vi "BRig_RT__Case_Exp__State_initTrial2__v17.vi"(0 "input_dataCurrent":u16[](array[numeric]), 1 "input_dataTrial":u16[][](array[numeric]), 3 "input_dataExp":u16[](array[numeric]), 6 "input_dataBlock":u16[][](array[numeric]), 8 "input_dataLC":u16[](array[numeric])) -> (7 "output_L_Wrong_Laser_l2":bool, 9 "output_L_Wrong_Event_l2":bool, 10 "output_L_Power_l1":dbl, 11 "output_L_Reward_Laser_l2":bool, 12 "output_L_Power_l2":dbl, 13 "output_L_Reward_Event_l2":bool, 14 "output_dataCurrent":u16[](array[numeric]), 15 "output_dataTrial":u16[][](array[numeric]), 16 "output_L_Reward_Event_l1":bool, 17 "output_L_Reward_Laser_l1":bool, 18 "output_L_Wrong_Event_l1":bool, 19 "output_L_Wrong_Laser_l1":bool)   [LabVIEW 2014]
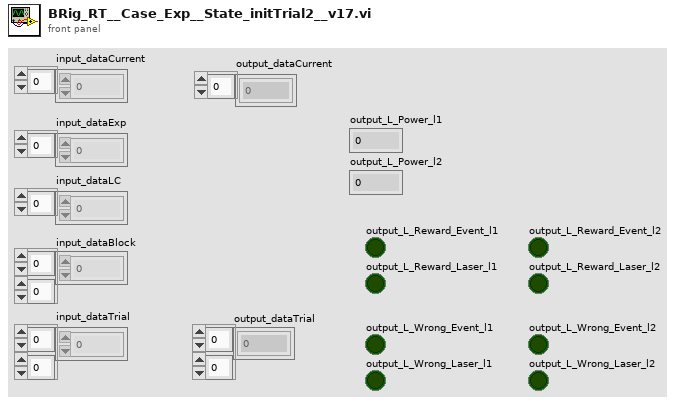
[diagram p1: front panel]
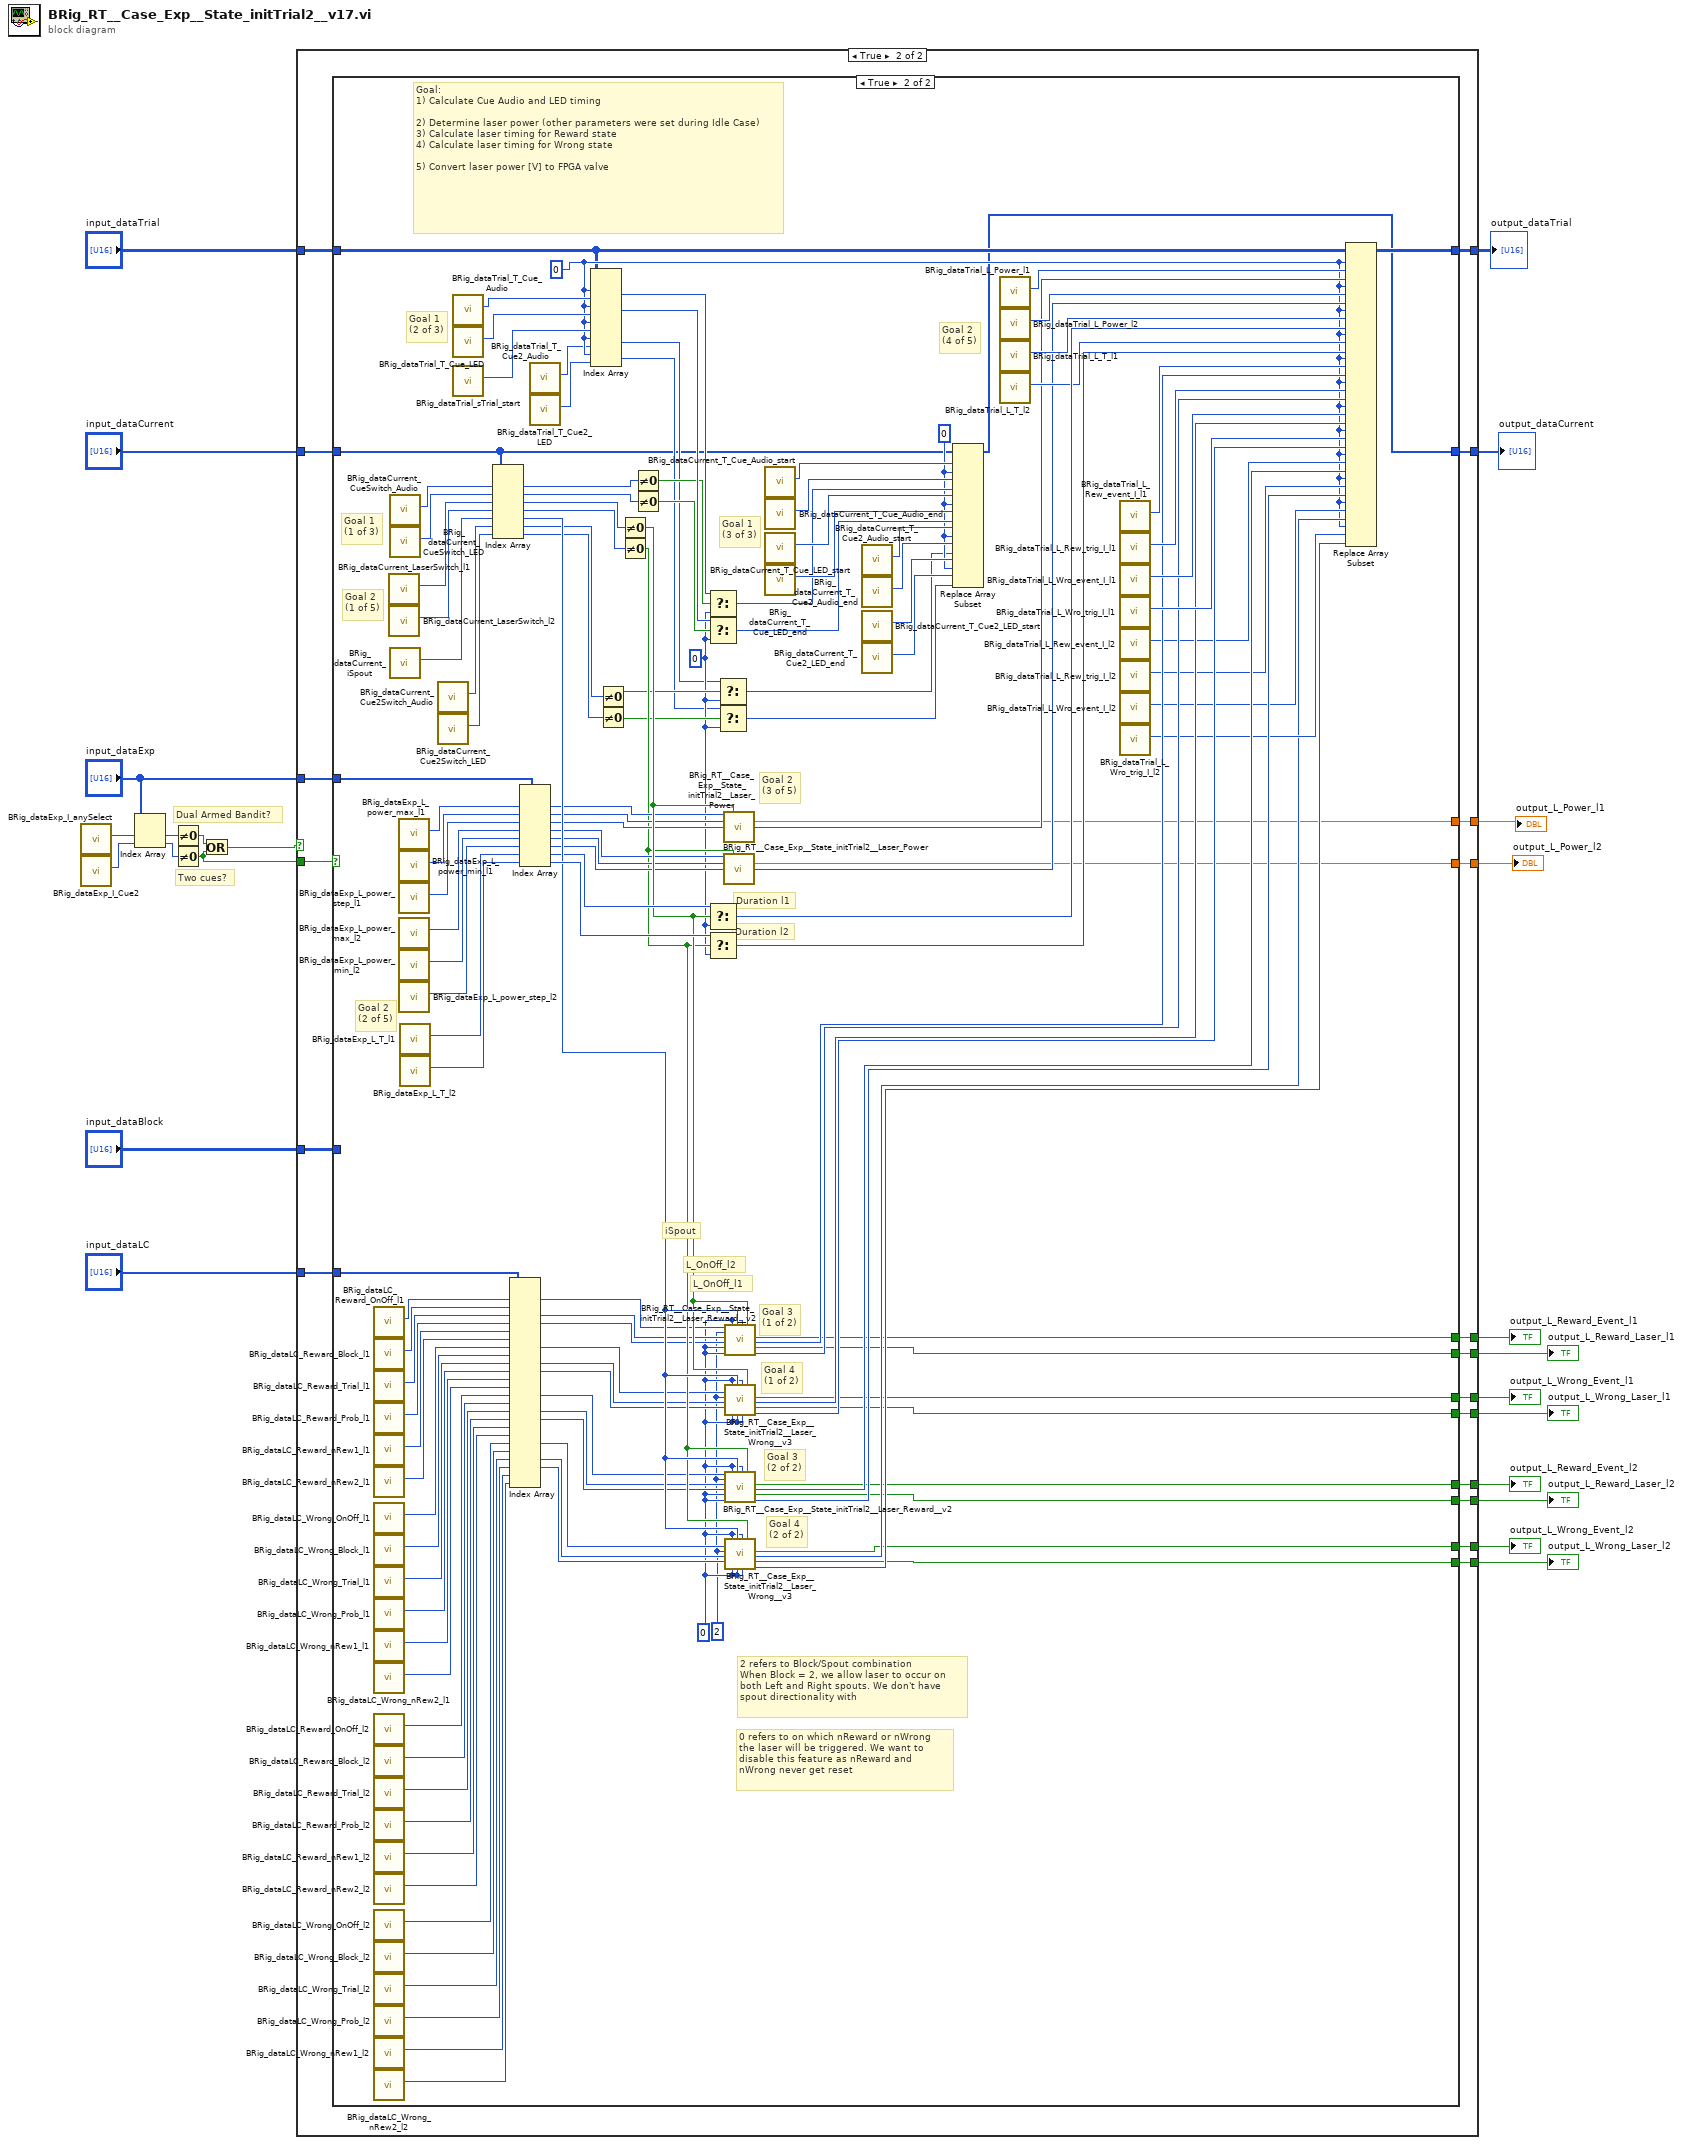
[diagram p0: block diagram]
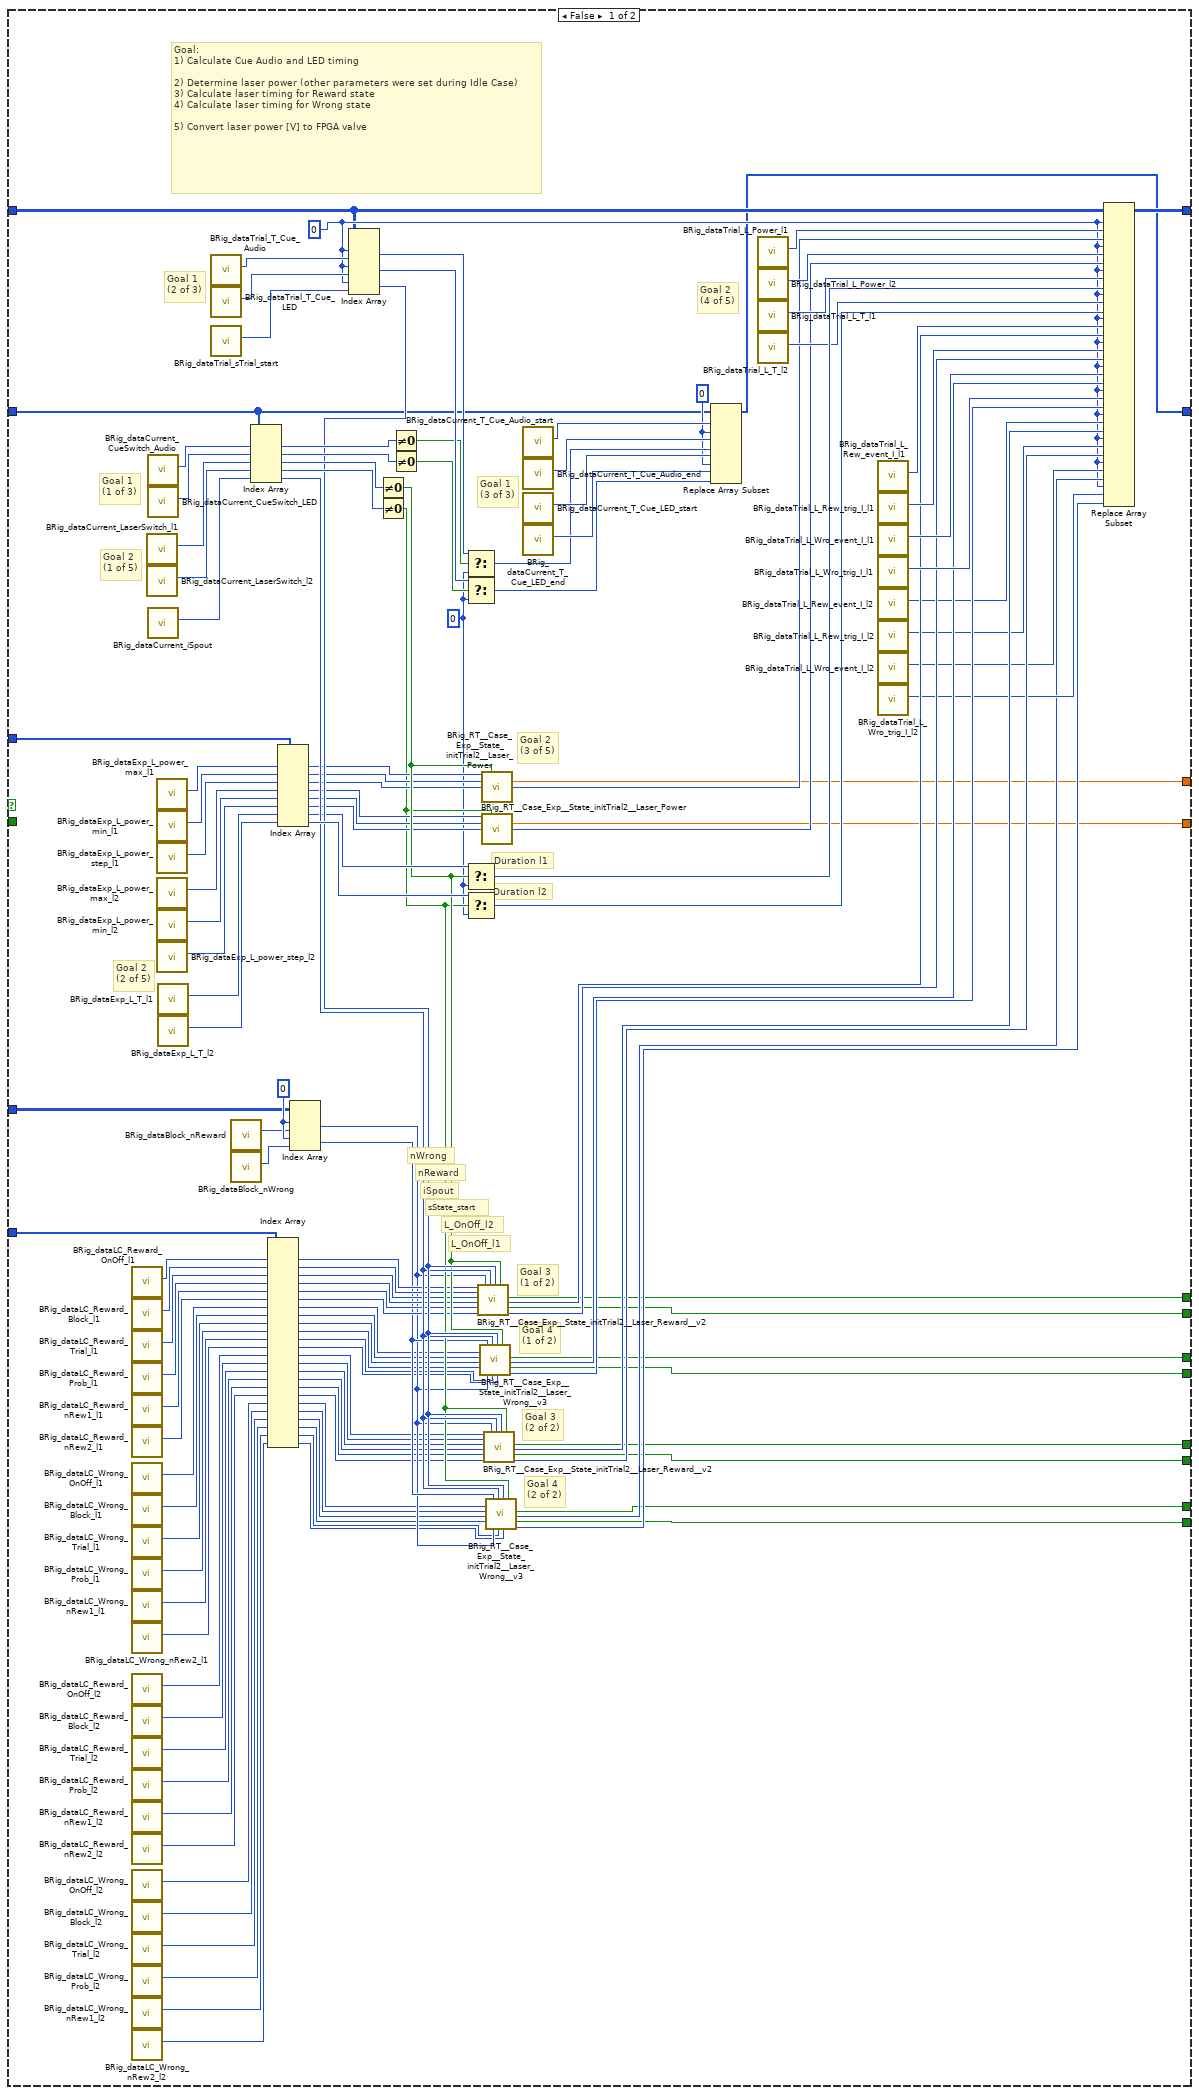
[diagram p2: hidden frame]
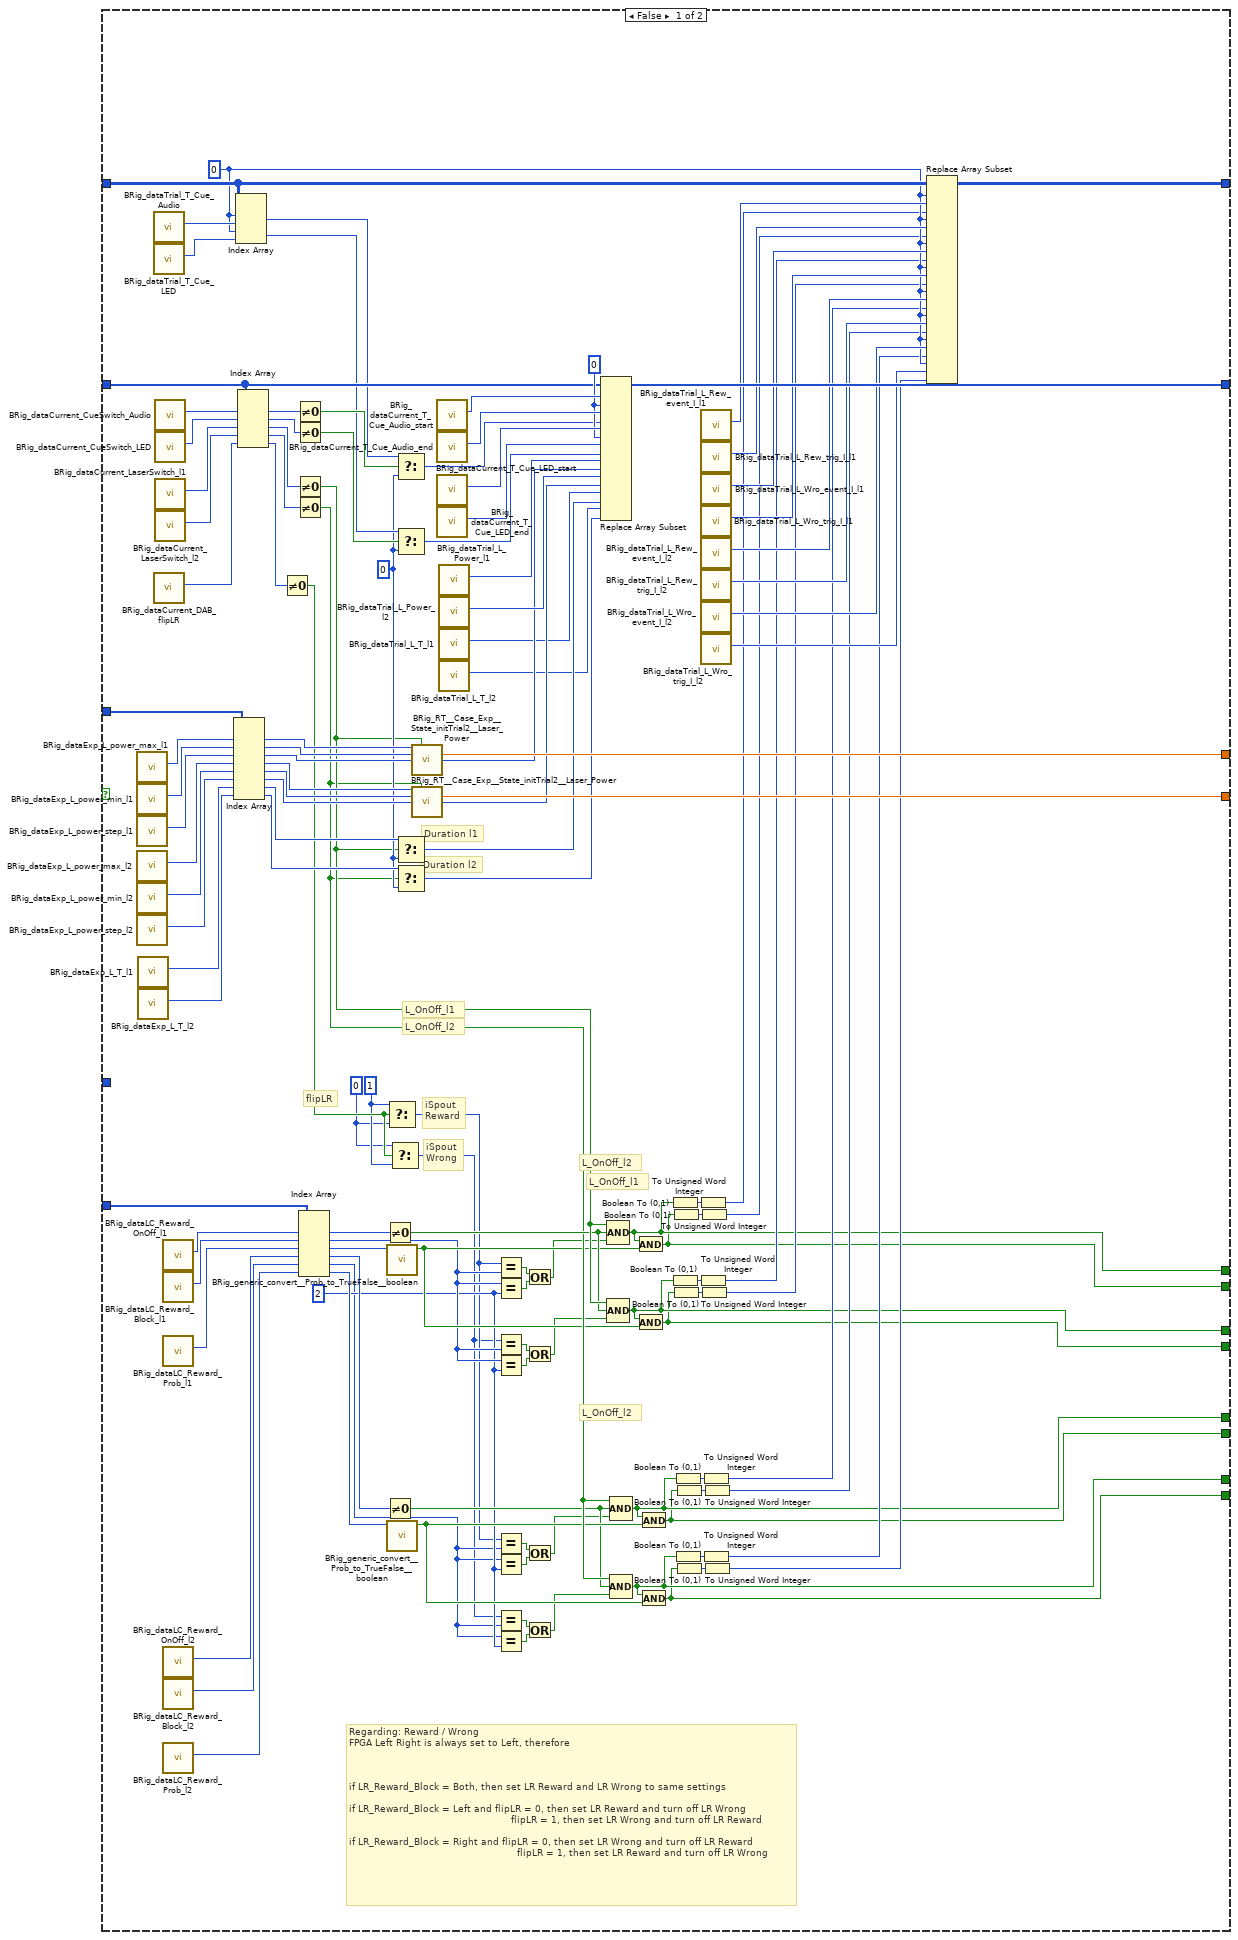
[diagram p3: hidden frame]
diagram:
  # "Two cues?"
  # "Dual Armed Bandit?"
  n1 = call "BRig_dataExp_I_anySelect.vi"() -> ("output_I_anySelect"=w9:i32)  [unwired: 11 in]
  n2 = call "BRig_dataExp_I_Cue2.vi"() -> ("output_I_Cue2"=w7:i32)  [unwired: 11 in]
  n3 = Index Array(array="input_dataExp", index #1=w9, index #2=w7) -> (element #1=w8:u16, element #2=w6:u16)
  n4 = Not Equal To 0?(x=w8) -> (x != 0?=w5:bool)
  n5 = Not Equal To 0?(x=w6) -> (x != 0?=w3:bool)
  n6 = Or(x=w5, y=w3) -> (x .or. y?=w4:bool)
  n7 = case shown="True" w4 {
    tunnel: [w41 w174] -> w24
    tunnel: "input_dataTrial" -> [w40 w175]
    tunnel: "input_dataCurrent" -> [w39 w181]
    tunnel: "input_dataExp" -> [w38 w179]
    tunnel: "input_dataBlock" -> [w37 w164]
    tunnel: "input_dataLC" -> [w36 w176]
    tunnel: [w35 w173] -> w19
    tunnel: [w34 w172] -> w18
    tunnel: [w33 w171] -> w17
    tunnel: [w32 w170] -> w16
    tunnel: [w31 w169] -> w15
    tunnel: [w30 w168] -> w14
    tunnel: [w29 w167] -> w13
    tunnel: [w28 w166] -> w12
    tunnel: [w27 w177] -> w11
    tunnel: [w26 w178] -> w10
    tunnel: [w25 w180] -> w1
    tunnel: w3 -> [_ w165]
    frame False {
      w89 = 0 ("disabled index (row)")
      w93 = 0
      w92 = u16 0 ("f")
      w91 = u16 0 ("new element/subarray")
      # "nWrong"
      # "nReward"
      # "L_OnOff_l2"
      # "Goal 2\n(3 of 5)"
      # "Goal 4\n(2 of 2)"
      # "Goal 4\n(1 of 2)"
      # "Goal 3\n(2 of 2)"
      # "Goal 3\n(1 of 2)"
      # "L_OnOff_l1"
      # "sState_start"
      # "iSpout"
      # "Goal 2\n(4 of 5)"
      # "Goal 2\n(2 of 5)"
      # "Duration l2"
      # "Duration l1"
      # "Goal 2\n(1 of 5)"
      # "Goal 1\n(3 of 3)"
      # "Goal 1\n(2 of 3)"
      # "Goal 1\n(1 of 3)"
      # "Goal:\n1) Calculate Cue Audio and LED timing\n\n2) Determine laser power (other parameters were set during Idle Case)\n3) Calculate laser timing for Reward state\n4) Calculate laser timing for Wrong state\n\n5) Convert laser power [V] to FPGA valve"
      n8 = call "BRig_dataLC_Reward_OnOff_l1.vi"() -> ("output_Reward_OnOff"=w130:i32)  [unwired: 11 in]
      n9 = call "BRig_dataLC_Reward_Block_l1.vi"() -> ("output_Reward_Block"=w129:i32)  [unwired: 11 in]
      n10 = call "BRig_dataLC_Reward_Trial_l1.vi"() -> ("output_Reward_Trial"=w128:i32)  [unwired: 11 in]
      n11 = call "BRig_dataLC_Reward_Prob_l1.vi"() -> ("output_Reward_Prob"=w127:i32)  [unwired: 11 in]
      n12 = call "BRig_dataLC_Reward_nRew1_l1.vi"() -> ("output_Reward_nRew1_l1"=w83:i32)  [unwired: 11 in]
      n13 = call "BRig_dataLC_Reward_nRew2_l1.vi"() -> ("output_Reward_nRew2_l1"=w82:i32)  [unwired: 11 in]
      n14 = call "BRig_dataLC_Wrong_OnOff_l1.vi"() -> ("output_Wrong_OnOff"=w79:i32)  [unwired: 11 in]
      n15 = call "BRig_dataLC_Wrong_Block_l1.vi"() -> ("output_Wrong_Block"=w78:i32)  [unwired: 11 in]
      n16 = call "BRig_dataLC_Wrong_Trial_l1.vi"() -> ("output_Wrong_Trial"=w77:i32)  [unwired: 11 in]
      n17 = call "BRig_dataLC_Wrong_Prob_l1.vi"() -> ("output_Wrong_Prob"=w76:i32)  [unwired: 11 in]
      n18 = call "BRig_dataLC_Wrong_nRew1_l1.vi"() -> ("output_Wrong_nRew1_l1"=w57:i32)  [unwired: 11 in]
      n19 = call "BRig_dataLC_Wrong_nRew2_l1.vi"() -> ("output_Wrong_nRew2_l1"=w56:i32)  [unwired: 11 in]
      n20 = call "BRig_dataLC_Reward_OnOff_l2.vi"() -> ("output_Reward_OnOff_l2"=w64:i32)  [unwired: 11 in]
      n21 = call "BRig_dataLC_Reward_Block_l2.vi"() -> ("output_Reward_Block_l2"=w65:i32)  [unwired: 11 in]
      n22 = call "BRig_dataLC_Reward_Trial_l2.vi"() -> ("output_Reward_Trial_l2"=w66:i32)  [unwired: 11 in]
      n23 = call "BRig_dataLC_Reward_Prob_l2.vi"() -> ("output_Reward_Prob_l2"=w67:i32)  [unwired: 11 in]
      n24 = call "BRig_dataLC_Reward_nRew1_l2.vi"() -> ("output_Reward_nRew1_l2"=w68:i32)  [unwired: 11 in]
      n25 = call "BRig_dataLC_Reward_nRew2_l2.vi"() -> ("output_Reward_nRew2_l2"=w69:i32)  [unwired: 11 in]
      n26 = call "BRig_dataLC_Wrong_OnOff_l2.vi"() -> ("output_Wrong_OnOff_l2"=w70:i32)  [unwired: 11 in]
      n27 = call "BRig_dataLC_Wrong_Block_l2.vi"() -> ("output_Wrong_Block_l2"=w71:i32)  [unwired: 11 in]
      n28 = call "BRig_dataLC_Wrong_Trial_l2.vi"() -> ("output_Wrong_Trial_l2"=w72:i32)  [unwired: 11 in]
      n29 = call "BRig_dataLC_Wrong_Prob_l2.vi"() -> ("output_Wrong_Prob_l2"=w73:i32)  [unwired: 11 in]
      n30 = call "BRig_dataLC_Wrong_nRew1_l2.vi"() -> ("output_Wrong_nRew1_l2"=w49:i32)  [unwired: 11 in]
      n31 = call "BRig_dataLC_Wrong_nRew2_l2.vi"() -> ("output_Wrong_nRew2_l2"=w48:i32)  [unwired: 11 in]
      n32 = call "BRig_dataCurrent_LaserSwitch_l1.vi"() -> ("output_LaserSwitch_l1"=w149:i32)  [unwired: 11 in]
      n33 = call "BRig_dataCurrent_LaserSwitch_l2.vi"() -> ("output_LaserSwitch_l2"=w148:i32)  [unwired: 11 in]
      n34 = call "BRig_dataCurrent_CueSwitch_Audio.vi"() -> ("output_CueSwitch_Audio"=w163:i32)  [unwired: 11 in]
      n35 = call "BRig_dataCurrent_CueSwitch_LED.vi"() -> ("output_CueSwitch_LED"=w162:i32)  [unwired: 11 in]
      n36 = call "BRig_dataCurrent_iSpout.vi"() -> ("output_iSpout"=w124:i32)  [unwired: 11 in]
      n37 = call "BRig_dataExp_L_power_max_l1.vi"() -> ("output_L_power_max_l1"=w147:i32)  [unwired: 11 in]
      n38 = call "BRig_dataExp_L_power_min_l1.vi"() -> ("output_L_power_min_l1"=w146:i32)  [unwired: 11 in]
      n39 = call "BRig_dataExp_L_power_step_l1.vi"() -> ("output_L_power_step_l1"=w145:i32)  [unwired: 11 in]
      n40 = call "BRig_dataExp_L_power_max_l2.vi"() -> ("output_L_power_max_l2"=w144:i32)  [unwired: 11 in]
      n41 = call "BRig_dataExp_L_power_min_l2.vi"() -> ("output_L_power_min_l2"=w143:i32)  [unwired: 11 in]
      n42 = call "BRig_dataExp_L_power_step_l2.vi"() -> ("output_L_power_step_l2"=w142:i32)  [unwired: 11 in]
      n43 = call "BRig_dataExp_L_T_l1.vi"() -> ("output_L_T_l1"=w141:i32)  [unwired: 11 in]
      n44 = call "BRig_dataExp_L_T_l2.vi"() -> ("output_L_T_l2"=w140:i32)  [unwired: 11 in]
      n45 = call "BRig_dataTrial_T_Cue_Audio.vi"() -> ("output_T_Cue_Audio"=w154:i32)  [unwired: 11 in]
      n46 = call "BRig_dataTrial_T_Cue_LED.vi"() -> ("output_T_Cue_LED"=w153:i32)  [unwired: 11 in]
      n47 = call "BRig_dataTrial_sTrial_start.vi"() -> ("output_sTrial_start"=w123:i32)  [unwired: 11 in]
      n48 = call "BRig_dataBlock_nReward.vi"() -> ("output_nReward"=w88:i32)  [unwired: 11 in]
      n49 = call "BRig_dataBlock_nWrong.vi"() -> ("output_nWrong"=w90:i32)  [unwired: 11 in]
      n50 = Index Array(array=w39, index #1=w163, index #2=w162, index #3=w149, index #4=w148, index #5=w124) -> (element #1=w157:u16, element #2=w156:u16, element #3=w126:u16, element #4=w125:u16, element #5=w121:u16)
      n51 = Index Array(array=w36, index #1=w130, index #2=w129, index #3=w128, index #4=w127, index #5=w83, index #6=w82, index #7=w79, index #8=w78, index #9=w77, index #10=w76, index #11=w57, index #12=w56, index #13=w64, index #14=w65, index #15=w66, index #16=w67, index #17=w68, index #18=w69, index #19=w70, index #20=w71, index #21=w72, index #22=w73, index #23=w49, index #24=w48) -> (element #1=w87:u16, element #2=w86:u16, element #3=w85:u16, element #4=w84:u16, element #5=w81:u16, element #6=w80:u16, element #7=w55:u16, element #8=w54:u16, element #9=w53:u16, element #10=w52:u16, element #11=w51:u16, element #12=w50:u16, element #13=w58:u16, element #14=w59:u16, element #15=w60:u16, element #16=w61:u16, element #17=w62:u16, element #18=w63:u16, element #19=w47:u16, element #20=w46:u16, element #21=w45:u16, element #22=w44:u16, element #23=w43:u16, element #24=w42:u16)
      n52 = Index Array(array=w38, index #1=w147, index #2=w146, index #3=w145, index #4=w144, index #5=w143, index #6=w142, index #7=w141, index #8=w140) -> (element #1=w102:u16, element #2=w101:u16, element #3=w100:u16, element #4=w98:u16, element #5=w97:u16, element #6=w96:u16, element #7=w104:u16, element #8=w137:u16)
      n53 = Index Array(array=w37, index (row) #1=w89, index (col) #1=w88, index (row) #2=w89, index (col) #2=w90) -> (element #1=w74:u16, element #2=w75:u16)
      n54 = Index Array(array=w40, index (row) #1=w93, index (col) #1=w154, index (row) #2=w93, index (col) #2=w153, index (row) #3=w93, index (col) #3=w123) -> (element #1=w152:u16, element #2=w151:u16, element #3=w122:u16)
      n55 = Not Equal To 0?(x=w126) -> (x != 0?=w103:bool)
      n56 = Not Equal To 0?(x=w125) -> (x != 0?=w95:bool)
      n57 = Not Equal To 0?(x=w157) -> (x != 0?=w139:bool)
      n58 = Not Equal To 0?(x=w156) -> (x != 0?=w138:bool)
      n59 = Select(t=w152, s=w139, f=w92) -> (s? t:f=w155:u16)
      n60 = Select(t=w151, s=w138, f=w92) -> (s? t:f=w150:u16)
      n61 = Select(t=w104, s=w103, f=w92) -> (s? t:f=w133:u16)
      n62 = Select(t=w137, s=w95, f=w92) -> (s? t:f=w131:u16)
      n63 = call "BRig_RT__Case_Exp__State_initTrial2__Laser_Reward__v2.vi"("input_L_OnOff"=w87, "input_L_Block"=w86, "input_L_Trial"=w85, "input_L_Probability"=w84, "input_L_nRew1"=w81, "input_L_nRew2"=w80, "input_nReward"=w74, "input_iSpout"=w121, "input_sState_start"=w122, "input_LaserSwitch"=w103) -> ("output_LR_Event"=w35:bool, "output_LR_Event_num"=w116:u16, "output_LR_Laser"=w34:bool, "output_LR_Laser_num"=w115:u16)  [unwired: 6 in]
      n64 = call "BRig_RT__Case_Exp__State_initTrial2__Laser_Wrong__v3.vi"("input_L_OnOff"=w55, "input_L_Block"=w54, "input_L_Trial"=w53, "input_L_Probability"=w52, "input_nWrong"=w75, "input_nReward"=w74, "input_iSpout"=w121, "input_L_nRew1"=w51, "input_sState_start"=w122, "input_L_nRew2"=w50, "input_LaserSwitch"=w103) -> ("output_LR_Event"=w33:bool, "output_LR_Event_num"=w114:u16, "output_LR_Laser"=w32:bool, "output_LR_Laser_num"=w113:u16)  [unwired: 5 in]
      n65 = call "BRig_RT__Case_Exp__State_initTrial2__Laser_Power.vi"("input_L_Power_max__x100"=w102, "input_LaserSwitch"=w103, "input_L_Power_min__x100"=w101, "input_L_Power_step__x100"=w100) -> ("output_L_Power"=w26:dbl, "output_L_Power_x100"=w99:u16)  [unwired: 10 in]
      n66 = call "BRig_RT__Case_Exp__State_initTrial2__Laser_Power.vi"("input_L_Power_max__x100"=w98, "input_LaserSwitch"=w95, "input_L_Power_min__x100"=w97, "input_L_Power_step__x100"=w96) -> ("output_L_Power"=w27:dbl, "output_L_Power_x100"=w94:u16)  [unwired: 10 in]
      n67 = call "BRig_RT__Case_Exp__State_initTrial2__Laser_Reward__v2.vi"("input_L_OnOff"=w58, "input_L_Block"=w59, "input_L_Trial"=w60, "input_L_Probability"=w61, "input_L_nRew1"=w62, "input_L_nRew2"=w63, "input_nReward"=w74, "input_iSpout"=w121, "input_sState_start"=w122, "input_LaserSwitch"=w95) -> ("output_LR_Event"=w31:bool, "output_LR_Event_num"=w111:u16, "output_LR_Laser"=w30:bool, "output_LR_Laser_num"=w109:u16)  [unwired: 6 in]
      n68 = call "BRig_RT__Case_Exp__State_initTrial2__Laser_Wrong__v3.vi"("input_L_OnOff"=w47, "input_L_Block"=w46, "input_L_Trial"=w45, "input_L_Probability"=w44, "input_nWrong"=w75, "input_nReward"=w74, "input_iSpout"=w121, "input_L_nRew1"=w43, "input_sState_start"=w122, "input_L_nRew2"=w42, "input_LaserSwitch"=w95) -> ("output_LR_Event"=w29:bool, "output_LR_Event_num"=w106:u16, "output_LR_Laser"=w28:bool, "output_LR_Laser_num"=w105:u16)  [unwired: 5 in]
      n69 = call "BRig_dataCurrent_T_Cue_Audio_start.vi"() -> ("output_T_Cue_Audio_start"=w161:i32)  [unwired: 11 in]
      n70 = call "BRig_dataCurrent_T_Cue_Audio_end.vi"() -> ("output_T_Cue_Audio_end"=w160:i32)  [unwired: 11 in]
      n71 = call "BRig_dataCurrent_T_Cue_LED_start.vi"() -> ("output_T_Cue_LED_start"=w159:i32)  [unwired: 11 in]
      n72 = call "BRig_dataCurrent_T_Cue_LED_end.vi"() -> ("output_T_Cue_LED_end"=w158:i32)  [unwired: 11 in]
      n73 = Replace Array Subset(array=w39, new element #1=w91, index #1=w161, new element #2=w155, index #2=w160, new element #3=w91, index #3=w159, new element #4=w150, index #4=w158) -> (w25:u16[])
      n74 = call "BRig_dataTrial_L_Power_l1.vi"() -> ("output_L_Power_l1"=w136:i32)  [unwired: 11 in]
      n75 = call "BRig_dataTrial_L_Power_l2.vi"() -> ("output_L_Power_l2"=w135:i32)  [unwired: 11 in]
      n76 = call "BRig_dataTrial_L_T_l1.vi"() -> ("output_L_T_l1"=w134:i32)  [unwired: 11 in]
      n77 = call "BRig_dataTrial_L_T_l2.vi"() -> ("output_L_T_l2"=w132:i32)  [unwired: 11 in]
      n78 = call "BRig_dataTrial_L_Rew_event_I_l1.vi"() -> ("output_L_Rew_event_I_l1"=w120:i32)  [unwired: 11 in]
      n79 = call "BRig_dataTrial_L_Rew_trig_I_l1.vi"() -> ("output_L_Rew_trig_I_l1"=w119:i32)  [unwired: 11 in]
      n80 = call "BRig_dataTrial_L_Wro_event_I_l1.vi"() -> ("output_L_Wro_event_I_l1"=w118:i32)  [unwired: 11 in]
      n81 = call "BRig_dataTrial_L_Wro_trig_I_l1.vi"() -> ("output_L_Wro_trig_I_l1"=w117:i32)  [unwired: 11 in]
      n82 = call "BRig_dataTrial_L_Rew_event_I_l2.vi"() -> ("output_L_Rew_event_I_l2"=w112:i32)  [unwired: 11 in]
      n83 = call "BRig_dataTrial_L_Rew_trig_I_l2.vi"() -> ("output_L_Rew_trig_I_l2"=w110:i32)  [unwired: 11 in]
      n84 = call "BRig_dataTrial_L_Wro_event_I_l2.vi"() -> ("output_L_Wro_event_I_l2"=w108:i32)  [unwired: 11 in]
      n85 = call "BRig_dataTrial_L_Wro_trig_I_l2.vi"() -> ("output_L_Wro_trig_I_l2"=w107:i32)  [unwired: 11 in]
      n86 = Replace Array Subset(array=w40, new element #1=w99, index (row) #1=w93, index (col) #1=w136, new element #2=w94, index (row) #2=w93, index (col) #2=w135, new element #3=w133, index (row) #3=w93, index (col) #3=w134, new element #4=w131, index (row) #4=w93, index (col) #4=w132, new element #5=w116, index (row) #5=w93, index (col) #5=w120, new element #6=w115, index (row) #6=w93, index (col) #6=w119, new element #7=w114, index (row) #7=w93, index (col) #7=w118, new element #8=w113, index (row) #8=w93, index (col) #8=w117, new element #9=w111, index (row) #9=w93, index (col) #9=w112, new element #10=w109, index (row) #10=w93, index (col) #10=w110, new element #11=w106, index (row) #11=w93, index (col) #11=w108, new element #12=w105, index (row) #12=w93, index (col) #12=w107) -> (w41:u16[][])
    }
    frame True {
      n87 = case shown="True" w165 {
        tunnel: w181 -> [w291 w323]
        tunnel: [w290 w309] -> w180
        tunnel: w179 -> [w267 w322]
        tunnel: [w265 w312] -> w178
        tunnel: [w264 w311] -> w177
        tunnel: w176 -> [w261 w321]
        tunnel: w175 -> [w244 w324]
        tunnel: [w243 w310] -> w174
        tunnel: [w189 w320] -> w173
        tunnel: [w188 w319] -> w172
        tunnel: [w187 w318] -> w171
        tunnel: [w186 w317] -> w170
        tunnel: [w185 w316] -> w169
        tunnel: [w184 w315] -> w168
        tunnel: [w183 w314] -> w167
        tunnel: [w182 w313] -> w166
        tunnel: w164 -> [_ _]
        frame False {
          w193 = u16 2 ("y")
          w238 = u16 1 ("input_sState_start")
          w237 = u16 0 ("input_sState_start")
          w266 = u16 0 ("f")
          w292 = u16 0 ("new element/subarray")
          w242 = 0
          # "L_OnOff_l2"
          # "iSpout\nWrong"
          # "iSpout\nReward"
          # "flipLR"
          # "Regarding: Reward / Wrong\nFPGA Left Right is always set to Left, therefore\n\n\n\nif LR_Reward_Block = Both, then set LR Reward and LR Wrong to same settings\n\nif LR_Reward_Block = Left and flipLR = 0, then set LR Reward and turn off LR Wrong\n                                                      flipLR = 1, then set LR Wrong and turn off LR Reward\n\nif LR_Reward_Block = Right and flipLR = 0, then set LR Wrong and turn off LR Reward\n                                                        flipLR = 1, then set LR Reward and turn off LR Wrong"
          # "L_OnOff_l1"
          # "L_OnOff_l2"
          # "L_OnOff_l2"
          # "L_OnOff_l1"
          # "Duration l2"
          # "Duration l1"
          n88 = call "BRig_dataExp_L_power_max_l1.vi"() -> ("output_L_power_max_l1"=w283:i32)  [unwired: 11 in]
          n89 = call "BRig_dataExp_L_power_min_l1.vi"() -> ("output_L_power_min_l1"=w282:i32)  [unwired: 11 in]
          n90 = call "BRig_dataExp_L_power_step_l1.vi"() -> ("output_L_power_step_l1"=w281:i32)  [unwired: 11 in]
          n91 = call "BRig_dataExp_L_power_max_l2.vi"() -> ("output_L_power_max_l2"=w280:i32)  [unwired: 11 in]
          n92 = call "BRig_dataExp_L_power_min_l2.vi"() -> ("output_L_power_min_l2"=w279:i32)  [unwired: 11 in]
          n93 = call "BRig_dataExp_L_power_step_l2.vi"() -> ("output_L_power_step_l2"=w278:i32)  [unwired: 11 in]
          n94 = call "BRig_dataExp_L_T_l1.vi"() -> ("output_L_T_l1"=w277:i32)  [unwired: 11 in]
          n95 = call "BRig_dataExp_L_T_l2.vi"() -> ("output_L_T_l2"=w276:i32)  [unwired: 11 in]
          n96 = call "BRig_dataTrial_T_Cue_Audio.vi"() -> ("output_T_Cue_Audio"=w306:i32)  [unwired: 11 in]
          n97 = call "BRig_dataTrial_T_Cue_LED.vi"() -> ("output_T_Cue_LED"=w305:i32)  [unwired: 11 in]
          n98 = call "BRig_dataCurrent_DAB_flipLR.vi"() -> ("output_DAB_flipLR"=w241:i32)  [unwired: 11 in]
          n99 = call "BRig_dataCurrent_CueSwitch_Audio.vi"() -> ("output_CueSwitch_Audio"=w304:i32)  [unwired: 11 in]
          n100 = call "BRig_dataCurrent_CueSwitch_LED.vi"() -> ("output_CueSwitch_LED"=w303:i32)  [unwired: 11 in]
          n101 = call "BRig_dataCurrent_LaserSwitch_l1.vi"() -> ("output_LaserSwitch_l1"=w302:i32)  [unwired: 11 in]
          n102 = call "BRig_dataCurrent_LaserSwitch_l2.vi"() -> ("output_LaserSwitch_l2"=w301:i32)  [unwired: 11 in]
          n103 = call "BRig_dataLC_Reward_OnOff_l1.vi"() -> ("output_Reward_OnOff"=w263:i32)  [unwired: 11 in]
          n104 = call "BRig_dataLC_Reward_Block_l1.vi"() -> ("output_Reward_Block"=w262:i32)  [unwired: 11 in]
          n105 = call "BRig_dataLC_Reward_Prob_l1.vi"() -> ("output_Reward_Prob"=w236:i32)  [unwired: 11 in]
          n106 = call "BRig_dataLC_Reward_OnOff_l2.vi"() -> ("output_Reward_OnOff_l2"=w235:i32)  [unwired: 11 in]
          n107 = call "BRig_dataLC_Reward_Block_l2.vi"() -> ("output_Reward_Block_l2"=w234:i32)  [unwired: 11 in]
          n108 = call "BRig_dataLC_Reward_Prob_l2.vi"() -> ("output_Reward_Prob_l2"=w233:i32)  [unwired: 11 in]
          n109 = Index Array(array=w267, index #1=w283, index #2=w282, index #3=w281, index #4=w280, index #5=w279, index #6=w278, index #7=w277, index #8=w276) -> (element #1=w273:u16, element #2=w272:u16, element #3=w271:u16, element #4=w270:u16, element #5=w269:u16, element #6=w268:u16, element #7=w274:u16, element #8=w275:u16)
          n110 = Index Array(array=w244, index (row) #1=w242, index (col) #1=w306, index (row) #2=w242, index (col) #2=w305) -> (element #1=w287:u16, element #2=w286:u16)
          n111 = Index Array(array=w291, index #1=w304, index #2=w303, index #3=w302, index #4=w301, index #5=w241) -> (element #1=w300:u16, element #2=w299:u16, element #3=w298:u16, element #4=w297:u16, element #5=w240:u16)
          n112 = Not Equal To 0?(x=w240) -> (x != 0?=w239:bool)
          n113 = Not Equal To 0?(x=w300) -> (x != 0?=w289:bool)
          n114 = Not Equal To 0?(x=w299) -> (x != 0?=w288:bool)
          n115 = Not Equal To 0?(x=w298) -> (x != 0?=w224:bool)
          n116 = Not Equal To 0?(x=w297) -> (x != 0?=w216:bool)
          n117 = Index Array(array=w261, index #1=w263, index #2=w262, index #3=w236, index #4=w235, index #5=w234, index #6=w233) -> (element #1=w232:u16, element #2=w205:u16, element #3=w231:u16, element #4=w199:u16, element #5=w191:u16, element #6=w197:u16)
          n118 = Not Equal To 0?(x=w232) -> (x != 0?=w223:bool)
          n119 = Not Equal To 0?(x=w199) -> (x != 0?=w196:bool)
          n120 = Select(t=w238, s=w239, f=w237) -> (s? t:f=w192:u16)
          n121 = call "BRig_generic_convert__Prob_to_TrueFalse__boolean.vi"("input_probability_u16"=w231) -> ("output_TF"=w211:bool)  [unwired: 10 in]
          n122 = call "BRig_generic_convert__Prob_to_TrueFalse__boolean.vi"("input_probability_u16"=w197) -> ("output_TF"=w198:bool)  [unwired: 10 in]
          n123 = Select(t=w237, s=w239, f=w238) -> (s? t:f=w190:u16)
          n124 = Select(t=w287, s=w289, f=w266) -> (s? t:f=w285:u16)
          n125 = Select(t=w286, s=w288, f=w266) -> (s? t:f=w284:u16)
          n126 = Select(t=w274, s=w224, f=w266) -> (s? t:f=w255:u16)
          n127 = Select(t=w275, s=w216, f=w266) -> (s? t:f=w253:u16)
          n128 = call "BRig_RT__Case_Exp__State_initTrial2__Laser_Power.vi"("input_L_Power_max__x100"=w273, "input_LaserSwitch"=w224, "input_L_Power_min__x100"=w272, "input_L_Power_step__x100"=w271) -> ("output_L_Power"=w265:dbl, "output_L_Power_x100"=w258:u16)  [unwired: 10 in]
          n129 = call "BRig_RT__Case_Exp__State_initTrial2__Laser_Power.vi"("input_L_Power_max__x100"=w270, "input_LaserSwitch"=w216, "input_L_Power_min__x100"=w269, "input_L_Power_step__x100"=w268) -> ("output_L_Power"=w264:dbl, "output_L_Power_x100"=w257:u16)  [unwired: 10 in]
          n130 = call "BRig_dataCurrent_T_Cue_Audio_start.vi"() -> ("output_T_Cue_Audio_start"=w296:i32)  [unwired: 11 in]
          n131 = call "BRig_dataCurrent_T_Cue_Audio_end.vi"() -> ("output_T_Cue_Audio_end"=w295:i32)  [unwired: 11 in]
          n132 = call "BRig_dataCurrent_T_Cue_LED_start.vi"() -> ("output_T_Cue_LED_start"=w294:i32)  [unwired: 11 in]
          n133 = call "BRig_dataCurrent_T_Cue_LED_end.vi"() -> ("output_T_Cue_LED_end"=w293:i32)  [unwired: 11 in]
          n134 = call "BRig_dataTrial_L_Power_l1.vi"() -> ("output_L_Power_l1"=w260:i32)  [unwired: 11 in]
          n135 = call "BRig_dataTrial_L_Power_l2.vi"() -> ("output_L_Power_l2"=w259:i32)  [unwired: 11 in]
          n136 = call "BRig_dataTrial_L_T_l1.vi"() -> ("output_L_T_l1"=w256:i32)  [unwired: 11 in]
          n137 = call "BRig_dataTrial_L_T_l2.vi"() -> ("output_L_T_l2"=w254:i32)  [unwired: 11 in]
          n138 = Equal?(x=w192, y=w205) -> (x = y?=w210:bool)
          n139 = Equal?(x=w205, y=w193) -> (x = y?=w209:bool)
          n140 = Equal?(x=w190, y=w205) -> (x = y?=w207:bool)
          n141 = Equal?(x=w205, y=w193) -> (x = y?=w206:bool)
          n142 = Equal?(x=w192, y=w191) -> (x = y?=w203:bool)
          n143 = Equal?(x=w191, y=w193) -> (x = y?=w202:bool)
          n144 = Equal?(x=w190, y=w191) -> (x = y?=w201:bool)
          n145 = Equal?(x=w191, y=w193) -> (x = y?=w200:bool)
          n146 = Or(x=w210, y=w209) -> (x .or. y?=w208:bool)
          n147 = Or(x=w207, y=w206) -> (x .or. y?=w204:bool)
          n148 = Or(x=w203, y=w202) -> (x .or. y?=w195:bool)
          n149 = Or(x=w201, y=w200) -> (x .or. y?=w194:bool)
          n150 = Replace Array Subset(array=w291, new element #1=w292, index #1=w296, new element #2=w285, index #2=w295, new element #3=w292, index #3=w294, new element #4=w284, index #4=w293, new element #5=w258, index #5=w260, new element #6=w257, index #6=w259, new element #7=w255, index #7=w256, new element #8=w253, index #8=w254) -> (w290:u16[])
          n151 = Compound Arithmetic op=AND(w224, w223, w208) -> (w189:bool)
          n152 = Compound Arithmetic op=AND(w224, w223, w204) -> (w187:bool)
          n153 = Compound Arithmetic op=AND(w216, w196, w195) -> (w185:bool)
          n154 = Compound Arithmetic op=AND(w216, w196, w194) -> (w183:bool)
          n155 = And(x=w189, y=w211) -> (x .and. y?=w188:bool)
          n156 = And(x=w187, y=w211) -> (x .and. y?=w186:bool)
          n157 = And(x=w185, y=w198) -> (x .and. y?=w184:bool)
          n158 = And(x=w183, y=w198) -> (x .and. y?=w182:bool)
          n159 = Boolean To (0,1)(Boolean=w189) -> (0, 1=w230:i16)
          n160 = Boolean To (0,1)(Boolean=w187) -> (0, 1=w226:i16)
          n161 = Boolean To (0,1)(Boolean=w188) -> (0, 1=w229:i16)
          n162 = Boolean To (0,1)(Boolean=w186) -> (0, 1=w225:i16)
          n163 = Boolean To (0,1)(Boolean=w185) -> (0, 1=w220:i16)
          n164 = Boolean To (0,1)(Boolean=w183) -> (0, 1=w218:i16)
          n165 = Boolean To (0,1)(Boolean=w184) -> (0, 1=w219:i16)
          n166 = Boolean To (0,1)(Boolean=w182) -> (0, 1=w217:i16)
          n167 = To Unsigned Word Integer(number=w230) -> (unsigned 16bit integer=w228:u16)
          n168 = To Unsigned Word Integer(number=w226) -> (unsigned 16bit integer=w222:u16)
          n169 = To Unsigned Word Integer(number=w229) -> (unsigned 16bit integer=w227:u16)
          n170 = To Unsigned Word Integer(number=w225) -> (unsigned 16bit integer=w221:u16)
          n171 = call "BRig_dataTrial_L_Rew_event_I_l1.vi"() -> ("output_L_Rew_event_I_l1"=w252:i32)  [unwired: 11 in]
          n172 = call "BRig_dataTrial_L_Rew_trig_I_l1.vi"() -> ("output_L_Rew_trig_I_l1"=w251:i32)  [unwired: 11 in]
          n173 = call "BRig_dataTrial_L_Wro_event_I_l1.vi"() -> ("output_L_Wro_event_I_l1"=w250:i32)  [unwired: 11 in]
          n174 = call "BRig_dataTrial_L_Wro_trig_I_l1.vi"() -> ("output_L_Wro_trig_I_l1"=w249:i32)  [unwired: 11 in]
          n175 = call "BRig_dataTrial_L_Rew_event_I_l2.vi"() -> ("output_L_Rew_event_I_l2"=w248:i32)  [unwired: 11 in]
          n176 = call "BRig_dataTrial_L_Rew_trig_I_l2.vi"() -> ("output_L_Rew_trig_I_l2"=w247:i32)  [unwired: 11 in]
          n177 = call "BRig_dataTrial_L_Wro_event_I_l2.vi"() -> ("output_L_Wro_event_I_l2"=w246:i32)  [unwired: 11 in]
          n178 = call "BRig_dataTrial_L_Wro_trig_I_l2.vi"() -> ("output_L_Wro_trig_I_l2"=w245:i32)  [unwired: 11 in]
          n179 = To Unsigned Word Integer(number=w220) -> (unsigned 16bit integer=w215:u16)
          n180 = To Unsigned Word Integer(number=w218) -> (unsigned 16bit integer=w213:u16)
          n181 = To Unsigned Word Integer(number=w219) -> (unsigned 16bit integer=w214:u16)
          n182 = To Unsigned Word Integer(number=w217) -> (unsigned 16bit integer=w212:u16)
          n183 = Replace Array Subset(array=w244, new element #1=w228, index (row) #1=w242, index (col) #1=w252, new element #2=w227, index (row) #2=w242, index (col) #2=w251, new element #3=w222, index (row) #3=w242, index (col) #3=w250, new element #4=w221, index (row) #4=w242, index (col) #4=w249, new element #5=w215, index (row) #5=w242, index (col) #5=w248, new element #6=w214, index (row) #6=w242, index (col) #6=w247, new element #7=w213, index (row) #7=w242, index (col) #7=w246, new element #8=w212, index (row) #8=w242, index (col) #8=w245) -> (w243:u16[][])
        }
        frame True {
          w307 = u16 2 ("input_L_Block")
          w308 = u16 0
          w375 = 0
          w366 = u16 0 ("f")
          w359 = u16 0 ("new element/subarray")
          # "0 refers to on which nReward or nWrong\nthe laser will be triggered. We want to\ndisable this feature as nReward and\nnWrong never get reset"
          # "2 refers to Block/Spout combination\nWhen Block = 2, we allow laser to occur on\nboth Left and Right spouts. We don't have\nspout directionality with"
          # "L_OnOff_l2"
          # "Goal 2\n(3 of 5)"
          # "Goal 4\n(2 of 2)"
          # "Goal 4\n(1 of 2)"
          # "Goal 3\n(2 of 2)"
          # "Goal 3\n(1 of 2)"
          # "L_OnOff_l1"
          # "iSpout"
          # "Goal 2\n(4 of 5)"
          # "Goal 2\n(2 of 5)"
          # "Duration l2"
          # "Duration l1"
          # "Goal 2\n(1 of 5)"
          # "Goal 1\n(3 of 3)"
          # "Goal 1\n(2 of 3)"
          # "Goal 1\n(1 of 3)"
          # "Goal:\n1) Calculate Cue Audio and LED timing\n\n2) Determine laser power (other parameters were set during Idle Case)\n3) Calculate laser timing for Reward state\n4) Calculate laser timing for Wrong state\n\n5) Convert laser power [V] to FPGA valve"
          n184 = call "BRig_dataLC_Reward_OnOff_l1.vi"() -> ("output_Reward_OnOff"=w411:i32)  [unwired: 11 in]
          n185 = call "BRig_dataLC_Reward_Block_l1.vi"() -> ("output_Reward_Block"=w410:i32)  [unwired: 11 in]
          n186 = call "BRig_dataLC_Reward_Trial_l1.vi"() -> ("output_Reward_Trial"=w409:i32)  [unwired: 11 in]
          n187 = call "BRig_dataLC_Reward_Prob_l1.vi"() -> ("output_Reward_Prob"=w408:i32)  [unwired: 11 in]
          n188 = call "BRig_dataLC_Reward_nRew1_l1.vi"() -> ("output_Reward_nRew1_l1"=w353:i32)  [unwired: 11 in]
          n189 = call "BRig_dataLC_Reward_nRew2_l1.vi"() -> ("output_Reward_nRew2_l1"=w352:i32)  [unwired: 11 in]
          n190 = call "BRig_dataLC_Wrong_OnOff_l1.vi"() -> ("output_Wrong_OnOff"=w351:i32)  [unwired: 11 in]
          n191 = call "BRig_dataLC_Wrong_Block_l1.vi"() -> ("output_Wrong_Block"=w350:i32)  [unwired: 11 in]
          n192 = call "BRig_dataLC_Wrong_Trial_l1.vi"() -> ("output_Wrong_Trial"=w349:i32)  [unwired: 11 in]
          n193 = call "BRig_dataLC_Wrong_Prob_l1.vi"() -> ("output_Wrong_Prob"=w348:i32)  [unwired: 11 in]
          n194 = call "BRig_dataLC_Wrong_nRew1_l1.vi"() -> ("output_Wrong_nRew1_l1"=w334:i32)  [unwired: 11 in]
          n195 = call "BRig_dataLC_Wrong_nRew2_l1.vi"() -> ("output_Wrong_nRew2_l1"=w333:i32)  [unwired: 11 in]
          n196 = call "BRig_dataLC_Reward_OnOff_l2.vi"() -> ("output_Reward_OnOff_l2"=w338:i32)  [unwired: 11 in]
          n197 = call "BRig_dataLC_Reward_Block_l2.vi"() -> ("output_Reward_Block_l2"=w339:i32)  [unwired: 11 in]
          n198 = call "BRig_dataLC_Reward_Trial_l2.vi"() -> ("output_Reward_Trial_l2"=w340:i32)  [unwired: 11 in]
          n199 = call "BRig_dataLC_Reward_Prob_l2.vi"() -> ("output_Reward_Prob_l2"=w341:i32)  [unwired: 11 in]
          n200 = call "BRig_dataLC_Reward_nRew1_l2.vi"() -> ("output_Reward_nRew1_l2"=w342:i32)  [unwired: 11 in]
          n201 = call "BRig_dataLC_Reward_nRew2_l2.vi"() -> ("output_Reward_nRew2_l2"=w343:i32)  [unwired: 11 in]
          n202 = call "BRig_dataLC_Wrong_OnOff_l2.vi"() -> ("output_Wrong_OnOff_l2"=w344:i32)  [unwired: 11 in]
          n203 = call "BRig_dataLC_Wrong_Block_l2.vi"() -> ("output_Wrong_Block_l2"=w345:i32)  [unwired: 11 in]
          n204 = call "BRig_dataLC_Wrong_Trial_l2.vi"() -> ("output_Wrong_Trial_l2"=w346:i32)  [unwired: 11 in]
          n205 = call "BRig_dataLC_Wrong_Prob_l2.vi"() -> ("output_Wrong_Prob_l2"=w347:i32)  [unwired: 11 in]
          n206 = call "BRig_dataLC_Wrong_nRew1_l2.vi"() -> ("output_Wrong_nRew1_l2"=w329:i32)  [unwired: 11 in]
          n207 = call "BRig_dataLC_Wrong_nRew2_l2.vi"() -> ("output_Wrong_nRew2_l2"=w328:i32)  [unwired: 11 in]
          n208 = call "BRig_dataCurrent_LaserSwitch_l1.vi"() -> ("output_LaserSwitch_l1"=w430:i32)  [unwired: 11 in]
          n209 = call "BRig_dataCurrent_LaserSwitch_l2.vi"() -> ("output_LaserSwitch_l2"=w429:i32)  [unwired: 11 in]
          n210 = call "BRig_dataCurrent_CueSwitch_Audio.vi"() -> ("output_CueSwitch_Audio"=w444:i32)  [unwired: 11 in]
          n211 = call "BRig_dataCurrent_CueSwitch_LED.vi"() -> ("output_CueSwitch_LED"=w443:i32)  [unwired: 11 in]
          n212 = call "BRig_dataCurrent_iSpout.vi"() -> ("output_iSpout"=w405:i32)  [unwired: 11 in]
          n213 = call "BRig_dataExp_L_power_max_l1.vi"() -> ("output_L_power_max_l1"=w428:i32)  [unwired: 11 in]
          n214 = call "BRig_dataExp_L_power_min_l1.vi"() -> ("output_L_power_min_l1"=w427:i32)  [unwired: 11 in]
          n215 = call "BRig_dataExp_L_power_step_l1.vi"() -> ("output_L_power_step_l1"=w426:i32)  [unwired: 11 in]
          n216 = call "BRig_dataExp_L_power_max_l2.vi"() -> ("output_L_power_max_l2"=w425:i32)  [unwired: 11 in]
          n217 = call "BRig_dataExp_L_power_min_l2.vi"() -> ("output_L_power_min_l2"=w424:i32)  [unwired: 11 in]
          n218 = call "BRig_dataExp_L_power_step_l2.vi"() -> ("output_L_power_step_l2"=w423:i32)  [unwired: 11 in]
          n219 = call "BRig_dataExp_L_T_l1.vi"() -> ("output_L_T_l1"=w422:i32)  [unwired: 11 in]
          n220 = call "BRig_dataExp_L_T_l2.vi"() -> ("output_L_T_l2"=w421:i32)  [unwired: 11 in]
          n221 = call "BRig_dataCurrent_Cue2Switch_Audio.vi"() -> ("output_Cue2Switch_Audio"=w372:i32)  [unwired: 11 in]
          n222 = call "BRig_dataCurrent_Cue2Switch_LED.vi"() -> ("output_Cue2Switch_LED"=w371:i32)  [unwired: 11 in]
          n223 = call "BRig_dataTrial_T_Cue_Audio.vi"() -> ("output_T_Cue_Audio"=w435:i32)  [unwired: 11 in]
          n224 = call "BRig_dataTrial_T_Cue_LED.vi"() -> ("output_T_Cue_LED"=w434:i32)  [unwired: 11 in]
          n225 = call "BRig_dataTrial_sTrial_start.vi"() -> ("output_sTrial_start"=w404:i32)  [unwired: 11 in]
          n226 = Index Array(array=w323, index #1=w444, index #2=w443, index #3=w430, index #4=w429, index #5=w405, index #6=w372, index #7=w371) -> (element #1=w438:u16, element #2=w437:u16, element #3=w407:u16, element #4=w406:u16, element #5=w403:u16, element #6=w370:u16, element #7=w369:u16)
          n227 = Index Array(array=w321, index #1=w411, index #2=w410, index #3=w409, index #4=w408, index #5=w353, index #6=w352, index #7=w351, index #8=w350, index #9=w349, index #10=w348, index #11=w334, index #12=w333, index #13=w338, index #14=w339, index #15=w340, index #16=w341, index #17=w342, index #18=w343, index #19=w344, index #20=w345, index #21=w346, index #22=w347, index #23=w329, index #24=w328) -> (element #1=w356:u16, element #3=w355:u16, element #4=w354:u16, element #7=w332:u16, element #9=w331:u16, element #10=w330:u16, element #13=w335:u16, element #15=w336:u16, element #16=w337:u16, element #19=w327:u16, element #21=w326:u16, element #22=w325:u16)  [unwired: 12 out]
          n228 = Index Array(array=w322, index #1=w428, index #2=w427, index #3=w426, index #4=w425, index #5=w424, index #6=w423, index #7=w422, index #8=w421) -> (element #1=w384:u16, element #2=w383:u16, element #3=w382:u16, element #4=w380:u16, element #5=w379:u16, element #6=w378:u16, element #7=w386:u16, element #8=w418:u16)
          n229 = call "BRig_dataTrial_T_Cue2_Audio.vi"() -> ("output_T_Cue2_Audio"=w374:i32)  [unwired: 11 in]
          n230 = call "BRig_dataTrial_T_Cue2_LED.vi"() -> ("output_T_Cue2_LED"=w373:i32)  [unwired: 11 in]
          n231 = Index Array(array=w324, index (row) #1=w375, index (col) #1=w435, index (row) #2=w375, index (col) #2=w434, index (row) #3=w375, index (col) #3=w404, index (row) #4=w375, index (col) #4=w374, index (row) #5=w375, index (col) #5=w373) -> (element #1=w433:u16, element #2=w432:u16, element #4=w365:u16, element #5=w364:u16)  [unwired: 1 out]
          n232 = Not Equal To 0?(x=w370) -> (x != 0?=w368:bool)
          n233 = Not Equal To 0?(x=w369) -> (x != 0?=w367:bool)
          n234 = Not Equal To 0?(x=w407) -> (x != 0?=w385:bool)
          n235 = Not Equal To 0?(x=w406) -> (x != 0?=w377:bool)
          n236 = Not Equal To 0?(x=w438) -> (x != 0?=w420:bool)
          n237 = Not Equal To 0?(x=w437) -> (x != 0?=w419:bool)
          n238 = Select(t=w433, s=w420, f=w366) -> (s? t:f=w436:u16)
          n239 = Select(t=w432, s=w419, f=w366) -> (s? t:f=w431:u16)
          n240 = Select(t=w386, s=w385, f=w366) -> (s? t:f=w414:u16)
          n241 = Select(t=w418, s=w377, f=w366) -> (s? t:f=w412:u16)
          n242 = Select(t=w365, s=w368, f=w366) -> (s? t:f=w358:u16)
          n243 = Select(t=w364, s=w367, f=w366) -> (s? t:f=w357:u16)
          n244 = call "BRig_RT__Case_Exp__State_initTrial2__Laser_Power.vi"("input_L_Power_max__x100"=w384, "input_LaserSwitch"=w385, "input_L_Power_min__x100"=w383, "input_L_Power_step__x100"=w382) -> ("output_L_Power"=w312:dbl, "output_L_Power_x100"=w381:u16)  [unwired: 10 in]
          n245 = call "BRig_RT__Case_Exp__State_initTrial2__Laser_Power.vi"("input_L_Power_max__x100"=w380, "input_LaserSwitch"=w377, "input_L_Power_min__x100"=w379, "input_L_Power_step__x100"=w378) -> ("output_L_Power"=w311:dbl, "output_L_Power_x100"=w376:u16)  [unwired: 10 in]
          n246 = call "BRig_RT__Case_Exp__State_initTrial2__Laser_Reward__v2.vi"("input_L_OnOff"=w356, "input_L_Block"=w307, "input_L_Trial"=w355, "input_L_Probability"=w354, "input_L_nRew1"=w308, "input_L_nRew2"=w308, "input_nReward"=w308, "input_iSpout"=w403, "input_sState_start"=w308, "input_LaserSwitch"=w385) -> ("output_LR_Event"=w320:bool, "output_LR_Event_num"=w398:u16, "output_LR_Laser"=w319:bool, "output_LR_Laser_num"=w397:u16)  [unwired: 6 in]
          n247 = call "BRig_RT__Case_Exp__State_initTrial2__Laser_Wrong__v3.vi"("input_L_OnOff"=w332, "input_L_Block"=w307, "input_L_Trial"=w331, "input_L_Probability"=w330, "input_nWrong"=w308, "input_nReward"=w308, "input_iSpout"=w403, "input_L_nRew1"=w308, "input_sState_start"=w308, "input_L_nRew2"=w308, "input_LaserSwitch"=w385) -> ("output_LR_Event"=w318:bool, "output_LR_Event_num"=w396:u16, "output_LR_Laser"=w317:bool, "output_LR_Laser_num"=w395:u16)  [unwired: 5 in]
          n248 = call "BRig_RT__Case_Exp__State_initTrial2__Laser_Reward__v2.vi"("input_L_OnOff"=w335, "input_L_Block"=w307, "input_L_Trial"=w336, "input_L_Probability"=w337, "input_L_nRew1"=w308, "input_L_nRew2"=w308, "input_nReward"=w308, "input_iSpout"=w403, "input_sState_start"=w308, "input_LaserSwitch"=w377) -> ("output_LR_Event"=w316:bool, "output_LR_Event_num"=w393:u16, "output_LR_Laser"=w315:bool, "output_LR_Laser_num"=w391:u16)  [unwired: 6 in]
          n249 = call "BRig_RT__Case_Exp__State_initTrial2__Laser_Wrong__v3.vi"("input_L_OnOff"=w327, "input_L_Block"=w307, "input_L_Trial"=w326, "input_L_Probability"=w325, "input_nWrong"=w308, "input_nReward"=w308, "input_iSpout"=w403, "input_L_nRew1"=w308, "input_sState_start"=w308, "input_L_nRew2"=w308, "input_LaserSwitch"=w377) -> ("output_LR_Event"=w314:bool, "output_LR_Event_num"=w388:u16, "output_LR_Laser"=w313:bool, "output_LR_Laser_num"=w387:u16)  [unwired: 5 in]
          n250 = call "BRig_dataCurrent_T_Cue_Audio_start.vi"() -> ("output_T_Cue_Audio_start"=w442:i32)  [unwired: 11 in]
          n251 = call "BRig_dataCurrent_T_Cue_Audio_end.vi"() -> ("output_T_Cue_Audio_end"=w441:i32)  [unwired: 11 in]
          n252 = call "BRig_dataCurrent_T_Cue_LED_start.vi"() -> ("output_T_Cue_LED_start"=w440:i32)  [unwired: 11 in]
          n253 = call "BRig_dataCurrent_T_Cue_LED_end.vi"() -> ("output_T_Cue_LED_end"=w439:i32)  [unwired: 11 in]
          n254 = call "BRig_dataCurrent_T_Cue2_Audio_start.vi"() -> ("output_T_Cue2_Audio_start"=w363:i32)  [unwired: 11 in]
          n255 = call "BRig_dataCurrent_T_Cue2_Audio_end.vi"() -> ("output_T_Cue2_Audio_end"=w362:i32)  [unwired: 11 in]
          n256 = call "BRig_dataCurrent_T_Cue2_LED_start.vi"() -> ("output_T_Cue2_LED_start"=w361:i32)  [unwired: 11 in]
          n257 = call "BRig_dataCurrent_T_Cue2_LED_end.vi"() -> ("output_T_Cue2_LED_end"=w360:i32)  [unwired: 11 in]
          n258 = Replace Array Subset(array=w323, new element #1=w359, index #1=w442, new element #2=w436, index #2=w441, new element #3=w359, index #3=w440, new element #4=w431, index #4=w439, new element #5=w359, index #5=w363, new element #6=w358, index #6=w362, new element #7=w359, index #7=w361, new element #8=w357, index #8=w360) -> (w309:u16[])
          n259 = call "BRig_dataTrial_L_Power_l1.vi"() -> ("output_L_Power_l1"=w417:i32)  [unwired: 11 in]
          n260 = call "BRig_dataTrial_L_Power_l2.vi"() -> ("output_L_Power_l2"=w416:i32)  [unwired: 11 in]
          n261 = call "BRig_dataTrial_L_T_l1.vi"() -> ("output_L_T_l1"=w415:i32)  [unwired: 11 in]
          n262 = call "BRig_dataTrial_L_T_l2.vi"() -> ("output_L_T_l2"=w413:i32)  [unwired: 11 in]
          n263 = call "BRig_dataTrial_L_Rew_event_I_l1.vi"() -> ("output_L_Rew_event_I_l1"=w402:i32)  [unwired: 11 in]
          n264 = call "BRig_dataTrial_L_Rew_trig_I_l1.vi"() -> ("output_L_Rew_trig_I_l1"=w401:i32)  [unwired: 11 in]
          n265 = call "BRig_dataTrial_L_Wro_event_I_l1.vi"() -> ("output_L_Wro_event_I_l1"=w400:i32)  [unwired: 11 in]
          n266 = call "BRig_dataTrial_L_Wro_trig_I_l1.vi"() -> ("output_L_Wro_trig_I_l1"=w399:i32)  [unwired: 11 in]
          n267 = call "BRig_dataTrial_L_Rew_event_I_l2.vi"() -> ("output_L_Rew_event_I_l2"=w394:i32)  [unwired: 11 in]
          n268 = call "BRig_dataTrial_L_Rew_trig_I_l2.vi"() -> ("output_L_Rew_trig_I_l2"=w392:i32)  [unwired: 11 in]
          n269 = call "BRig_dataTrial_L_Wro_event_I_l2.vi"() -> ("output_L_Wro_event_I_l2"=w390:i32)  [unwired: 11 in]
          n270 = call "BRig_dataTrial_L_Wro_trig_I_l2.vi"() -> ("output_L_Wro_trig_I_l2"=w389:i32)  [unwired: 11 in]
          n271 = Replace Array Subset(array=w324, new element #1=w381, index (row) #1=w375, index (col) #1=w417, new element #2=w376, index (row) #2=w375, index (col) #2=w416, new element #3=w414, index (row) #3=w375, index (col) #3=w415, new element #4=w412, index (row) #4=w375, index (col) #4=w413, new element #5=w398, index (row) #5=w375, index (col) #5=w402, new element #6=w397, index (row) #6=w375, index (col) #6=w401, new element #7=w396, index (row) #7=w375, index (col) #7=w400, new element #8=w395, index (row) #8=w375, index (col) #8=w399, new element #9=w393, index (row) #9=w375, index (col) #9=w394, new element #10=w391, index (row) #10=w375, index (col) #10=w392, new element #11=w388, index (row) #11=w375, index (col) #11=w390, new element #12=w387, index (row) #12=w375, index (col) #12=w389) -> (w310:u16[][])
        }
      }
    }
  }
  "output_dataTrial" <- w24
  "output_L_Reward_Event_l1" <- w19
  "output_L_Wrong_Event_l1" <- w17
  "output_L_Reward_Event_l2" <- w15
  "output_L_Wrong_Event_l2" <- w13
  "output_L_Reward_Laser_l1" <- w18
  "output_L_Wrong_Laser_l1" <- w16
  "output_L_Reward_Laser_l2" <- w14
  "output_L_Wrong_Laser_l2" <- w12
  "output_L_Power_l2" <- w11
  "output_L_Power_l1" <- w10
  "output_dataCurrent" <- w1
